vi "PPMS.getAngle.vi"(8 "error in (no error)":errorcluster, 11 "instrument.PPMS":refnum<class "instrument.PPMS.lvclass">) -> (0 "error out":errorcluster, 2 "Angle (°)":dbl, 3 "instrument.PPMS out":refnum<class "instrument.PPMS.lvclass">)   [LabVIEW 2019, in "instrument.PPMS.lvclass"]
uses:
  instrument.PPMS.lvclass
  instrument.PPMS.lvclass/instrument.PPMS.ctl
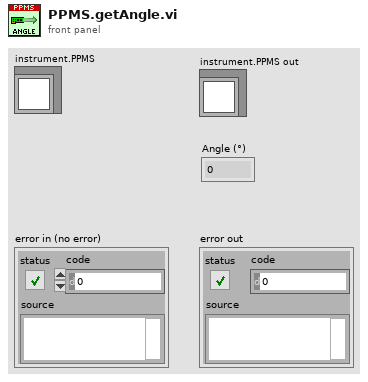
[diagram p1: front panel]
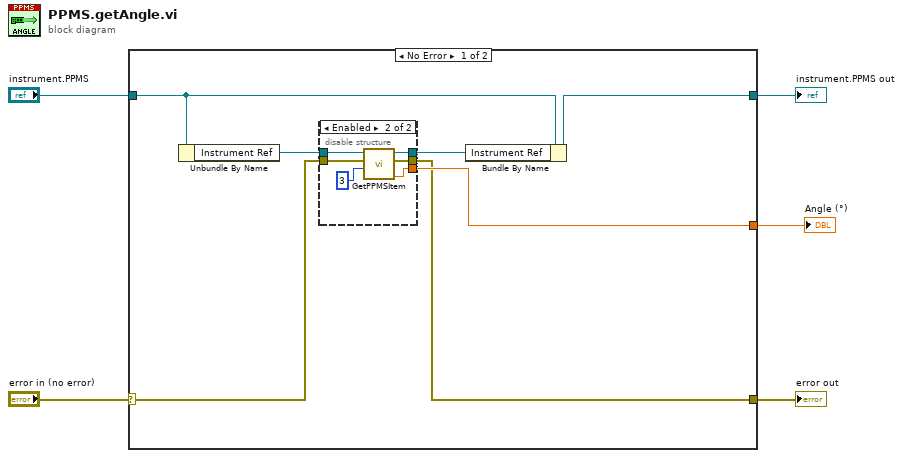
[diagram p0: block diagram]
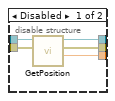
[diagram p2: hidden frame]
diagram:
  n1 = case shown="No Error" "error in (no error)" {
    selector: "error in (no error)" -> [w8 w25]
    tunnel: [w6 w25] -> w5
    tunnel: "instrument.PPMS" -> [w11 w24]
    tunnel: [w12 w24] -> w2
    tunnel: [w7 _] -> w1
    frame No Error {
      n2 = Unbundle By Name(w11) -> ("Instrument Ref"=w10:refnum<k24>)
      n3 = disable-structure shown="Enabled" {
        disable-tunnel: w10 -> [w17 w23]
        disable-tunnel: [w16 w19] -> w9
        disable-tunnel: w8 -> [w15 w21]
        disable-tunnel: [w14 w18] -> w7
        disable-tunnel: [w13 w20] -> w6
        frame Disabled {
          n4 = call "GetPosition.vi"("error in (no error)"=w15, "Instrument Ref In"=w17) -> ("Position"=w14:dbl, "error out"=w13:errorcluster, "Instrument Ref Out"=w16:refnum<k24>)  [unwired: 2 in, 1 out]
        }
        frame Enabled {
          n5 = call "GetPPMSItem.vi"("Channel"=3, "error in (no error)"=w21, "Instrument Ref In"=w23) -> ("Result"=w18:dbl, "error out"=w20:errorcluster, "Instrument Ref Out"=w19:refnum<k24>)  [unwired: 1 in, 1 out]
        }
      }
      n6 = Bundle By Name(cluster=w11, "Instrument Ref"=w9) -> (w12:refnum<class "instrument.PPMS.lvclass">)
    }
    frame Error {
    }
  }
  "Angle (°)" <- w1
  "error out" <- w5
  "instrument.PPMS out" <- w2
